vi "sendMessage.vi"(8 "error in (no error)":errorcluster, 9 "message_end":T1, 10 "Message":string, 11 "tcpDevice in":refnum<class "tcpDevice.lvclass">) -> (0 "error out":errorcluster, 3 "tcpDevice out":refnum<class "tcpDevice.lvclass">)   [LabVIEW 2016, in "tcpDevice.lvclass"]
uses:
  tcpDevice.lvclass
  typedefs/messageEnd.ctl
  tcpDevice.lvclass/tcpDevice.ctl
  ts_labview_tcp/TCPClient/TCPClient.lvclass
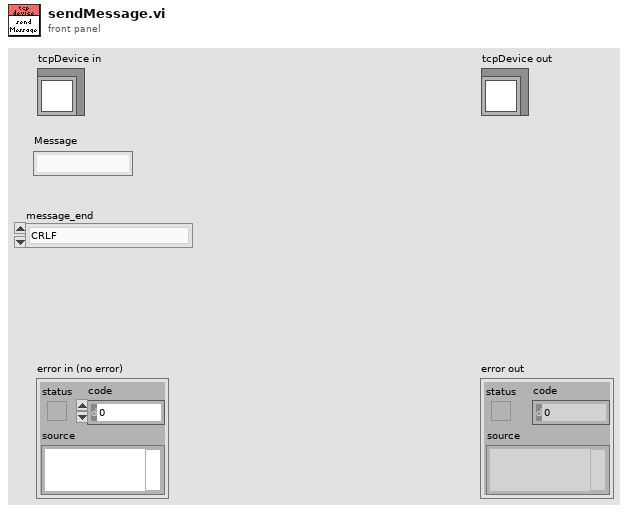
[diagram p1: front panel]
types:
  T1 = typedef "messageEnd.ctl" = enum16{"CRLF"}
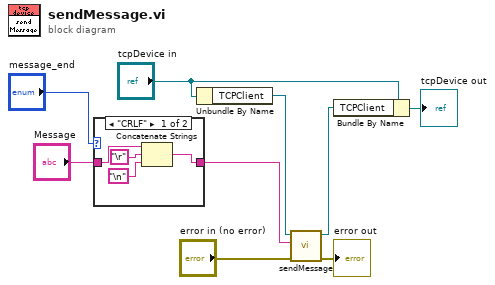
[diagram p0: block diagram]
diagram:
  n1 = case shown="\"CRLF\"" "message_end" {
    tunnel: "Message" -> [w12 w14]
    tunnel: [w13 w14] -> w2
    frame "CRLF" {
      n2 = Concatenate Strings(w12, "\r", "\n") -> (w13:string)
    }
    frame Default {
    }
  }
  n3 = Unbundle By Name("tcpDevice in") -> ("TCPClient"=w9:refnum<class "TCPClient.lvclass">)
  n4 = call-dynamic "sendMessage.vi"("error in (no error)"="error in (no error)", "String"=w2, "TCPClient in"=w9) -> ("error out"=→"error out":errorcluster, "TCPClient out"=w8:refnum<class "TCPClient.lvclass">)  [unwired: 7 in]
  n5 = Bundle By Name(cluster="tcpDevice in", "TCPClient"=w8) -> (→"tcpDevice out":refnum<class "tcpDevice.lvclass">)
